vi "ExSubSetupCascade.vi"(2 "error in (no error)":errorcluster, 3 "OverLap Mode":bool, 4 "Camera Handle":u32) -> (0 "error out":errorcluster, 1 "Camera Handle":u32)   [LabVIEW 2010]
panel:
  # "ExSubSetupCascade:\nThis Sub VI sets up the skips, cleans, and shutter parameters.\nThis should be changed to suit the camera you are using."
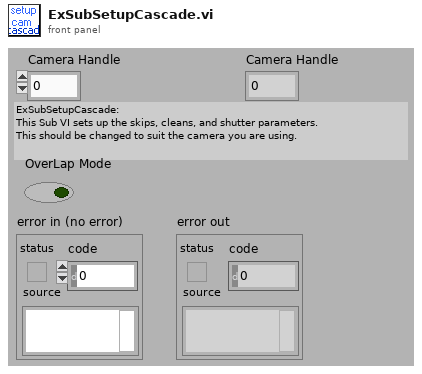
[diagram p1: front panel]
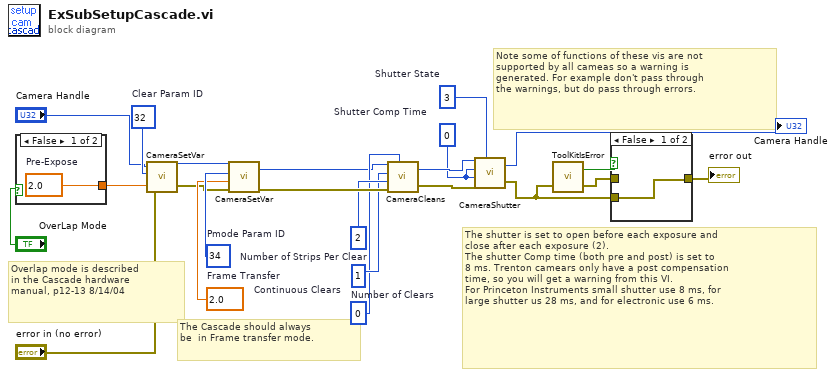
[diagram p0: block diagram]
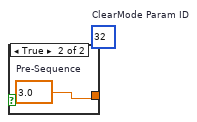
[diagram p2: hidden frame]
diagram:
  w2 = u32 3  # Shutter State
  w3 = u32 0  # Shutter Comp Time
  w9 = u32 1  # Number of Clears
  w10 = u32 2  # Number of Strips Per Clear
  w8 = u32 0  # Continuous Clears
  w16 = 2.0  # Frame Transfer
  w18 = 32  # Clear Param ID
  w17 = 34  # Pmode Param ID
  # "Overlap mode is described \nin the Cascade hardware \nmanual, p12-13 8/14/04"
  # "The Cascade should always\nbe  in Frame transfer mode."
  # "Note some of functions of these vis are not \nsupported by all cameas so a warning is \ngenerated. For example don't pass through \nthe warnings, but do pass through errors."
  # "The shutter is set to open before each exposure and\nclose after each exposure (2).\nThe shutter Comp time (both pre and post) is set to \n8 ms. Trenton camears only have a post compensation \ntime, so you will get a warning from this VI.\nFor Princeton Instruments small shutter use 8 ms, for \nlarge shutter us 28 ms, and for electronic use 6 ms."
  n1 = case shown="False" "OverLap Mode" {
    tunnel: [w24 w25] -> w19
    frame False {
      w24 = 2.0  # Pre-Expose
    }
    frame True {
      w25 = 3.0  # Pre-Sequence
      (unwired) 32  # ClearMode Param ID
    }
  }
  n2 = call <userlib>:"CameraSetVar.vi"("error in"="error in (no error)", "Value"=w19, "Parameter ID"=w18, "Camera Handle"="Camera Handle") -> ("error out"=w15:errorcluster, "CameraHandle"=w14:u32)
  n3 = call <userlib>:"CameraSetVar.vi"("error in"=w15, "Value"=w16, "Parameter ID"=w17, "Camera Handle"=w14) -> ("error out"=w11:errorcluster, "CameraHandle"=w1:u32)
  n4 = call <userlib>:"CameraCleans.vi"("Camera Handle"=w1, "Number of Clears"=w9, "Number of Strips Per Clear"=w10, "error in"=w11, "Continuous Clears"=w8) -> ("Camera Handle"=w6:u32, "error out"=w7:errorcluster)
  n5 = call <userlib>:"CameraShutter.vi"("Camera Handle"=w6, "Shutter Comp Time: Pre Open"=w3, "Shutter Comp Time: Post Open"=w3, "error in"=w7, "Shutter State"=w2) -> ("Camera Handle"=→"Camera Handle":u32, "error out"=w5:errorcluster)
  n6 = call <userlib>:"ToolKitIsError.vi"("error in"=w5) -> ("error out"=w22:errorcluster, "Error Flag"=w23:bool)  [unwired: 1 in]
  n7 = case shown="False" w23 {
    tunnel: w22 -> [_ w27]
    tunnel: [w26 w27] -> w21
    tunnel: w5 -> [w26 _]
    frame False {
    }
    frame True {
    }
  }
  "error out" <- w21
